vi "update_mode.vi"(8 "error in (no error)":errorcluster, 11 "mode":T1) -> (0 "error out":errorcluster)   [LabVIEW 2015, in "lv-recipe-machine.lvlib"]
uses:
  lv-recipe-machine.lvlib
  _controls/mode.ctl
  _controls/automatic_state.ctl
  _controls/manual_state.ctl
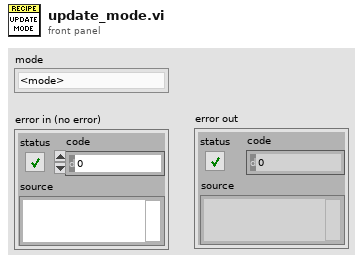
[diagram p1: front panel]
types:
  T1 = typedef "lv-recipe-machine.lvlib/mode.ctl" = enum16{"<mode>", "manual", "automatic", "<null>"}
  T2 = typedef "lv-recipe-machine.lvlib/automatic_state.ctl" = enum16{"<automatic_state>", "failed", "idle", "running", "paused", "stopped", "<null>"}
  T3 = typedef "lv-recipe-machine.lvlib/manual_state.ctl" = enum16{"<manual_state>", "failed", "action", "running", "idle", "<null>"}
  T4 = typedef "lv-recipe-machine.lvlib/references.ctl" = cluster{"semaphore":T5, "input_queue":refnum<queue>, "output_queue":refnum<queue>, "transition_queue":refnum<queue>, "data_dvr":refnum<data-value>, "stop_notifier":refnum<notifier>, "change_in_event":refnum<user-event>, "change_out_event":refnum<user-event>, "status_event":refnum<user-event>}
  T5 = typedef "Semaphore RefNum" = refnum<k1>
  T6 = typedef "lv-recipe-machine.lvlib/data.ctl" = cluster{"configuration":T7, "working":cluster{"recipe_data":T8}}
  T7 = typedef "lv-recipe-machine.lvlib/configuration.ctl" = cluster{"change_in_timeout_ms":i32}
  T8 = typedef "lv-recipe-machine.lvlib/recipe_data.ctl" = cluster{"mode":T1, "manual_state":T3, "automatic_state":T2, "previous_automatic_state":T2, "error":errorcluster, "timer []":T9[], "manual":cluster{"step_action":string, "data":variant, "actions":variant}, "automatic":cluster{"data":variant, "steps":variant, "criteria":variant, "transition":string, "index":i32, "step_launched":bool, "recipe []":T10[]}}
  T9 = typedef "lv-recipe-machine.lvlib/timer.ctl" = cluster{"elapsed_time":dbl, "previous_time":dbl}
  T10 = typedef "lv-recipe-machine.lvlib/recipe_step.ctl" = cluster{"step":string, "data":variant}
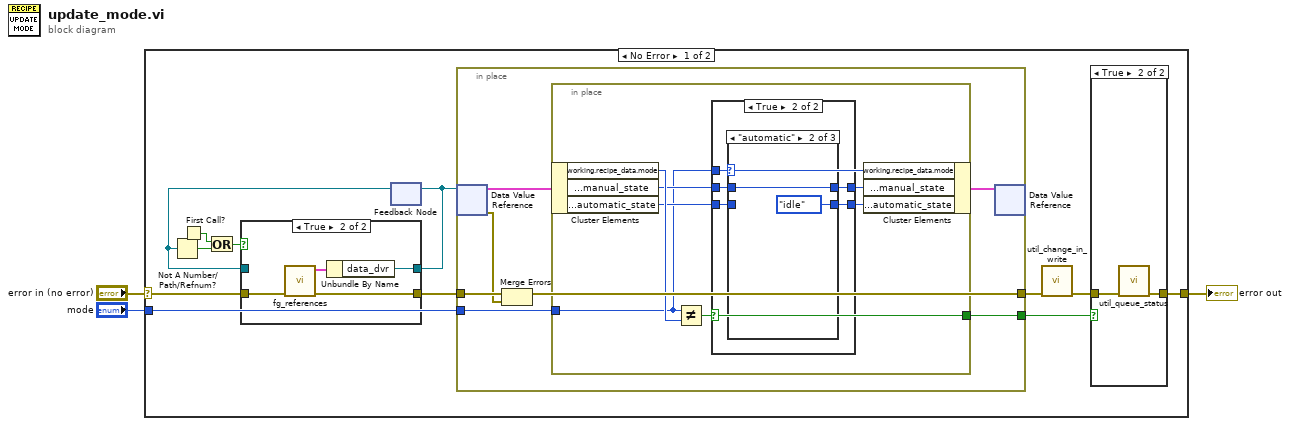
[diagram p0: block diagram]
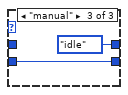
[diagram p5: hidden frame]
diagram:
  n1 = case shown="No Error" "error in (no error)" {
    selector: "error in (no error)" -> [w5 w52]
    tunnel: [w12 w52] -> w2
    tunnel: "mode" -> [w15 _]
    frame No Error {
      n2 = First Call?() -> (First Call?: T/F=w9:bool)
      n3 = feedback #1() -> (w8:refnum<data-value>)  [unwired: 1 in]
      n4 = Not A Number/Path/Refnum?(number/path/refnum=w8) -> (NaN/Path/Refnum?=w10:bool)
      n5 = Or(x=w9, y=w10) -> (x .or. y?=w7:bool)
      n6 = case shown="True" w7 {
        tunnel: w5 -> [w16 w21]
        tunnel: [w16 w20] -> w4
        tunnel: [w17 w18] -> w6
        tunnel: w8 -> [w17 _]
        frame False {
        }
        frame True {
          n7 = call "fg_references.vi"("error in (no error)"=w21) -> ("error out"=w20:errorcluster, "references out"=w19:T4)  [unwired: 9 in]
          n8 = Unbundle By Name(w19) -> ("data_dvr"=w18:refnum<data-value>)
        }
      }
      n9 = feedback-in #1(w6) -> ()
      n10 = in-place {
        in-place-border: [w26] -> w14
        in-place-border: w4 -> [w28]
        in-place-border: w15 -> [w23]
        in-place-border: [w22] -> w11
        n11 = in-place-dvr #2(w6) -> (w25:T6, w27:errorcluster)
        n12 = Merge Errors(w28, w27) -> (w26:errorcluster)
        n13 = in-place {
          in-place-border: w23 -> [w29]
          in-place-border: [w34] -> w22
          n14 = in-place-cluster #3(w25) -> ("working.recipe_data.mode"=w35:T1, "working.recipe_data.manual_state"=w33:T3, "working.recipe_data.automatic_state"=w31:T2)
          n15 = Not Equal?(x=w29, y=w35) -> (x != y?=w34:bool)
          n16 = case shown="True" w34 {
            tunnel: w33 -> [w37 w41]
            tunnel: [w37 w40] -> w32
            tunnel: w31 -> [w36 w39]
            tunnel: [w36 w38] -> w30
            tunnel: w29 -> [_ w42]
            frame False {
            }
            frame True {
              n17 = case shown="\"automatic\"" w42 {
                tunnel: w41 -> [w44 w46 _]
                tunnel: [w44 w46 manual_state."idle" ("manual_state")] -> w40
                tunnel: w39 -> [w43 _ w47]
                tunnel: [w43 automatic_state."idle" ("automatic_state") w47] -> w38
                frame Default {
                }
                frame "automatic" {
                }
                frame "manual" {
                }
              }
            }
          }
          n18 = in-place-cluster #3("working.recipe_data.mode"=w29, "working.recipe_data.manual_state"=w32, "working.recipe_data.automatic_state"=w30) -> (w24:T6)
        }
        n19 = in-place-dvr #2(w24) -> ()  [unwired: 2 out]
      }
      n20 = call "util_change_in_write.vi"("error in (no error)"=w14) -> ("error out"=w13:errorcluster)  [unwired: 10 in]
      n21 = case shown="True" w11 {
        tunnel: w13 -> [w49 w51]
        tunnel: [w49 w50] -> w12
        frame False {
        }
        frame True {
          n22 = call "util_queue_status.vi"("error in (no error)"=w51) -> ("error out"=w50:errorcluster)  [unwired: 10 in]
        }
      }
    }
    frame Error {
    }
  }
  "error out" <- w2
